vi "solar Pack.vi"(8 "error in (no error)":errorcluster, 9 "TLM_DATA in":variant, 10 "TLM in":string, 11 "solar in":refnum<class "solar.lvclass">) -> (0 "error out":errorcluster, 1 "TLM_DATA out":variant, 2 "TLM out":string, 3 "solar out":refnum<class "solar.lvclass">)   [LabVIEW 2018, in "solar.lvclass"]
doc: "Handle packing custom target messages."
uses:
  solar.lvclass
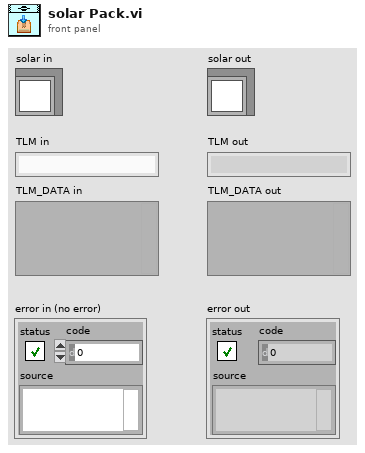
[diagram p1: front panel]
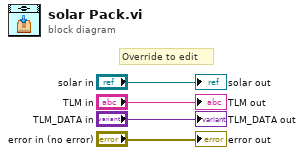
[diagram p0: block diagram]
diagram:
  # "Override to edit"
  "error out" <- "error in (no error)"
  "solar out" <- "solar in"
  "TLM out" <- "TLM in"
  "TLM_DATA out" <- "TLM_DATA in"
